vi "ConfigureDlg.vi"(8 "error in (no error)":errorcluster, 11 "C37.118 PMU in":refnum<class "C37.118 Sim.lvclass">) -> (0 "error out":errorcluster, 2 "Changed":bool, 3 "C37.118 PMU out":refnum<class "C37.118 Sim.lvclass">)   [LabVIEW 2018, in "SensorPlugins.lvlib" / "C37.118 Sim.lvclass"]
uses:
  C37.118 Sim.lvclass
  X:/Projects/PMUCal/Modules/Sensor/SensorPlugins/PmuBaseClass/PmuBase.lvclass
  C:/Program Files (x86)/National Instruments/LabVIEW 2018/user.lib/NIST/BaseClasses/BasePlugin_class/BasePlugin.lvclass
  PmuBaseClass/Typedef/PmuConfig.ctl
  PmuBaseClass/Typedef/ePhases.ctl
  PmuBaseClass/PmuBase.lvclass/PmuBase.ctl
  C37.118 Sim.lvclass/C37.118 Sim.ctl
  <userlib>/NIST/BaseClasses/BasePlugin_class/BasePlugin.lvclass/BasePlugin.ctl
  FGen/MemberClasses/FunctionBaseClass/FunctionBase.lvclass
  PmuBaseClass/Accessors/Read PmuConfig.vi
  PmuBaseClass/Accessors/Read PhaseArray.vi
  Accessors/Read FunctionIniFilePath.vi
  PmuBaseClass/Accessors/Write PmuConfig.vi
  PmuBaseClass/Accessors/Write PhaseArray.vi
  <userlib>/NIST/BaseClasses/BasePlugin_class/Accessors/Read PluginIniFilePath.vi
  <userlib>/NIST/BaseClasses/BasePlugin_class/Accessors/Write PluginIniFilePath.vi
  Accessors/Write Function.vi
  Accessors/Write FunctionIniFilePath.vi
  Accessors/Read Function.vi
  <vilib>/Utility/error.llb/Error Cluster From Error Code.vi
  <vilib>/ErrorRing/Error Ring.xnode
  <vilib>/Utility/config.llb/NI_LVConfig.lvlib
  <userlib>/NIST/NISTErrorLib/NISTErrorLib.lvlib
  <userlib>/NIST/BaseClasses/Object_class/BaseObject.lvclass
  PmuBaseClass/PmuBase.lvclass
panel:
  in  "btnSaveAs":bool
  in  "FunctionIniFilePath":path
  in  "btnFuncConfig":bool
  in  "btnCancel":bool
  in  "BtnDone":bool
  in  "PhaseArray":T1[](array[typedef])=[enum."VA", enum."VB", enum."VC", enum."V+", enum."IA", enum."IB", enum."IC", enum."I+"]
  in  "PmuConfig":T2={"Class"=enum."M", "Fs"=60, "F0"=60, "FSamp"=60, "SettlingTime"=0.0, "T0"=0.0}
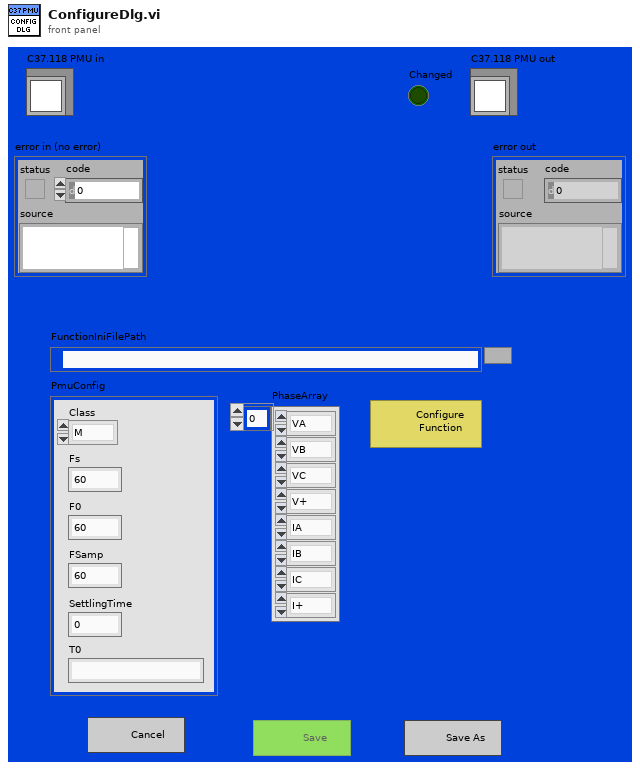
[diagram p1: front panel]
types:
  T1 = typedef "SensorPlugins.lvlib/PmuBase.lvclass/ePhases.ctl" = enum16{"VA", "VB", "VC", "V+", "IA", "IB", "IC", "I+", "none"}
  T2 = typedef "SensorPlugins.lvlib/PmuBase.lvclass/PmuConfig.ctl" = cluster{"Class":enum16{"M", "P"}, "Fs":i32, "F0":i32, "FSamp":i32, "SettlingTime":dbl, "T0":ext}
  T3 = enum8{"Enabled", "Disabled", "Disabled and Grayed Out"}
  T4 = enum32{"Invalid", "Standard", "Closed", "Hidden", "Minimized", "Maximized"}
  T5 = enum32{"Invalid", "Default", "Floating", "Floating/Auto-Hide", "Modal"}
  T6 = typedef "NI_LVConfig.lvlib/Config Data RefNum.ctl" = refnum<k1>
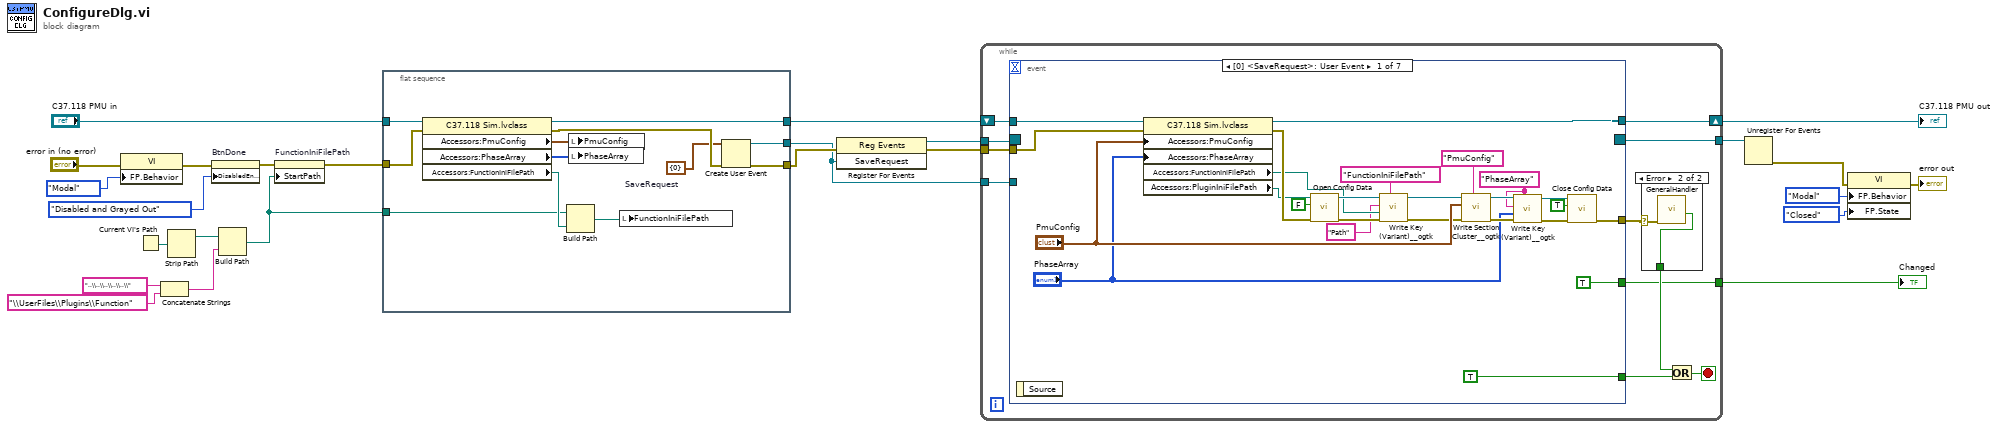
[diagram p0: block diagram]
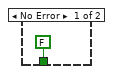
[diagram p2: hidden frame]
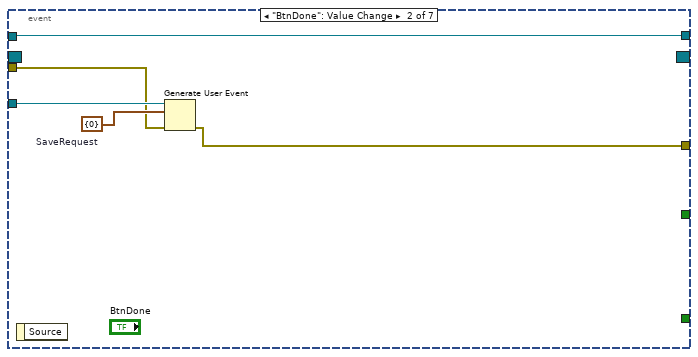
[diagram p3: hidden frame]
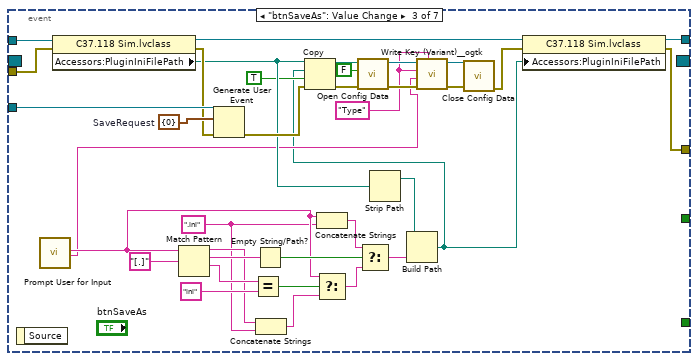
[diagram p4: hidden frame]
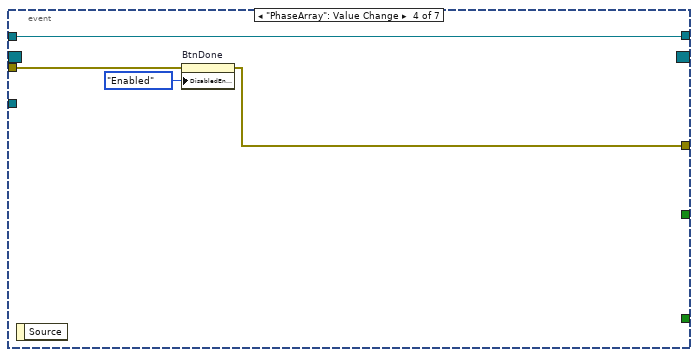
[diagram p5: hidden frame]
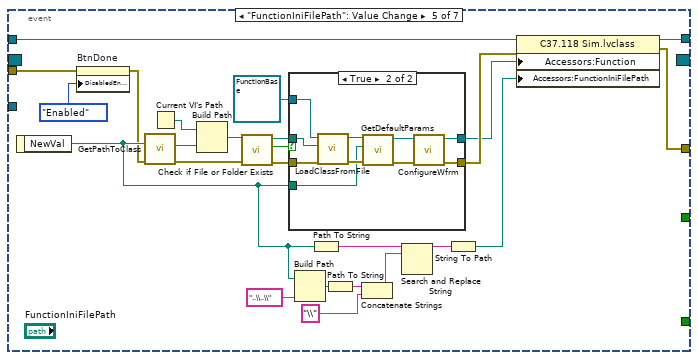
[diagram p6: hidden frame]
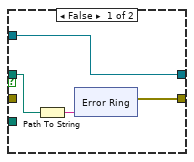
[diagram p7: hidden frame]
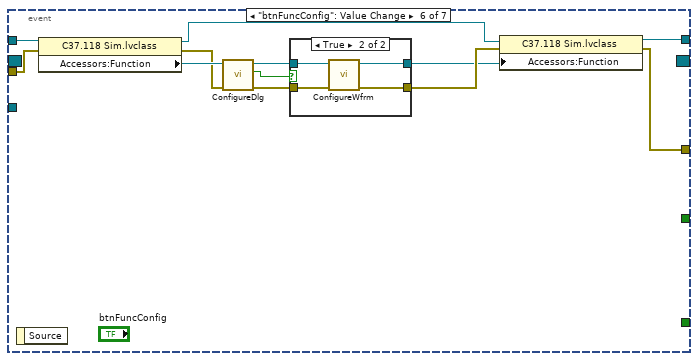
[diagram p8: hidden frame]
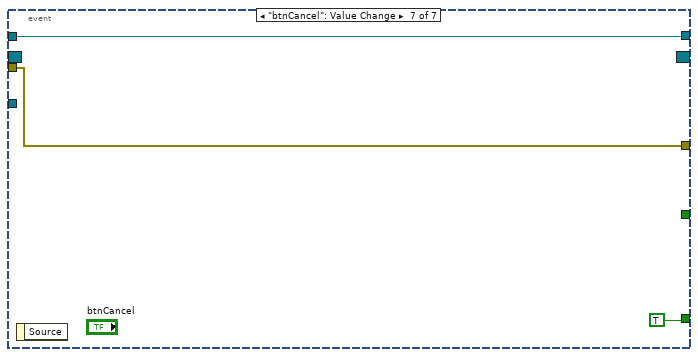
[diagram p10: hidden frame]
diagram:
  n1 = property class="VI"(error in="error in (no error)", "FP.Behavior"=T5."Modal" ("Front Panel Window:Behavior")) -> (error out=w16:errorcluster)  [unwired: 1 in, 1 out]
  n2 = Current VI's Path() -> (path=w11:path)
  n3 = Concatenate Strings("..\\..\\..\\..\\..\\", "\\UserFiles\\Plugins\\Function" ("name or relative path")) -> (w13:string)
  n4 = Strip Path(path=w11) -> (stripped path=w14:path)  [unwired: 1 out]
  n5 = property on="BtnDone" class="Bool"(error in=w16, "DisabledEnum"=T3."Disabled and Grayed Out" ("Disabled")) -> (error out=w9:errorcluster)  [unwired: 1 in, 1 out]
  n6 = Build Path(base path=w14, name or relative path=w13) -> (appended path=w7:path)
  n7 = property on="FunctionIniFilePath" class="Path"(error in=w9, "StartPath"=w7) -> (error out=w8:errorcluster)  [unwired: 1 in, 1 out]
  n8 = flat-sequence {
    tunnel: "C37.118 PMU in" -> [w37]
    tunnel: [w36] -> w23
    tunnel: [w29] -> w6
    tunnel: w8 -> [w35]
    tunnel: w7 -> [w31]
    tunnel: [w26] -> w4
    frame #0 {
      w27 = cluster{"Num":i32} {"Num"=0}  # SaveRequest
      n9 = property class="C37.118 Sim.lvclass"(reference=w37, error in=w35) -> (reference out=w36:refnum<class "C37.118 Sim.lvclass">, error out=w28:errorcluster, "Accessors:PmuConfig"=w34:T2, "Accessors:PhaseArray"=w33:T1[], "Accessors:FunctionIniFilePath"=w32:path)
      n10 = Build Path(base path=w31, name or relative path=w32) -> (appended path=w30:path)
      n11 = local write "PmuConfig"(w34) -> ()
      n12 = local write "PhaseArray"(w33) -> ()
      n13 = local write "FunctionIniFilePath"(w30) -> ()
      n14 = Create User Event(user event datatype=w27, error in=w28) -> (user event=w26:refnum<user-event>, error out=w29:errorcluster)
    }
  }
  n15 = register-events(error in=w6, w4) -> (reference out=w3:refnum<event-registration>, error out=w5:errorcluster)  [unwired: 1 in]
  n16 = while {
    shift-right: [w46] -> w24
    shift-left: w23 -> [w48]
    tunnel: w5 -> [w47]
    tunnel: [w41] -> w21
    tunnel: w4 -> [w40]
    tunnel: w3 -> [w39]
    tunnel: [w38] -> w2
    stop <- w42 stop-if-true
    n17 = event shown="[0] <SaveRequest>: User Event" {
      selector: w39 -> [_ _ _ _ _ _ _]
      dyn-events: [_ _ _ _ _ _ _] -> w38
      timeout: _ -> [_ _ _ _ _ _ _]
      tunnel: w48 -> [w76 w77 w105 w120 w131 w179 w188]
      tunnel: w47 -> [w74 w79 w102 w121 w124 w178 w187]
      tunnel: [w63 w78 w83 w118 w125 w173 w187] -> w43
      tunnel: [TRUE _ _ _ _ _ TRUE] -> w45
      tunnel: [w73 w77 w103 w120 w126 w174 w188] -> w46
      tunnel: [TRUE _ _ _ _ _ _] -> w41
      tunnel: w40 -> [_ w81 w101 _ _ _ _]
      event User Event {
        w62 = "PhaseArray" ("section (optional)")
        n18 = event-data() -> ()  [unwired: 1 in, 1 out]
        n19 = property class="C37.118 Sim.lvclass"(reference=w76, error in=w74, "Accessors:PmuConfig"="PmuConfig", "Accessors:PhaseArray"="PhaseArray") -> (reference out=w73:refnum<class "C37.118 Sim.lvclass">, error out=w71:errorcluster, "Accessors:FunctionIniFilePath"=w53:path, "Accessors:PluginIniFilePath"=w58:path)
        n20 = call <vilib>:"Open Config Data.vi"("error in (no error)"=w71, "create file if necessary (T)"=FALSE, "configuration file path"=w58) -> ("error out"=w56:errorcluster, "refnum"=w70:T6)  [unwired: 6 in, 1 out]
        n21 = call <userlib>:"Write Key (Variant)__ogtk.vi"("section"="FunctionIniFilePath", "error in (no error)"=w56, "key-value"=w53, "key (optional)"="Path", "refnum"=w70) -> ("error out"=w55:errorcluster, "refnum out"=w57:T6)  [unwired: 5 in]
        n22 = call <userlib>:"Write Section Cluster__ogtk.vi"("section (optional)"="PmuConfig", "error in (no error)"=w55, "Section Formatted Cluster"="PmuConfig", "refnum"=w57) -> ("error out"=w67:errorcluster, "dup refnum"=w66:T6)  [unwired: 6 in]
        n23 = call <userlib>:"Write Key (Variant)__ogtk.vi"("section"=w62, "error in (no error)"=w67, "key-value"="PhaseArray", "key (optional)"=w62, "refnum"=w66) -> ("error out"=w60:errorcluster, "refnum out"=w61:T6)  [unwired: 5 in]
        n24 = call <vilib>:"Close Config Data.vi"("error in (no error)"=w60, "write file if changed (T)"=TRUE, "refnum"=w61) -> ("error out"=w63:errorcluster)  [unwired: 7 in, 1 out]
      }
      event "BtnDone": Value Change {
        w80 = cluster{"Num":i32} {"Num"=0}  # SaveRequest
        n25 = event-data() -> ()  [unwired: 1 in, 1 out]
        n26 = Generate User Event(user event=w81, event data cluster=w80, error in=w79) -> (error out=w78:errorcluster)  [unwired: 1 in, 1 out]
      }
      event "btnSaveAs": Value Change {
        w82 = "Type"
        w100 = cluster{"Num":i32} {"Num"=0}  # SaveRequest
        w86 = ".ini" ("string")
        n27 = event-data() -> ()  [unwired: 1 in, 1 out]
        n28 = call "Prompt User for Input"() -> ("File Name"=w106:string, "PluginType Name"=w87:string)  [unwired: 16 in, 2 out]
        n29 = property class="C37.118 Sim.lvclass"(reference=w105, error in=w102) -> (reference out=w104:refnum<class "C37.118 Sim.lvclass">, error out=w99:errorcluster, "Accessors:PluginIniFilePath"=w90:path)
        n30 = Match Pattern(string=w106, regular expression="[.]" ("string")) -> (before substring=w113:string, match substring=w115:string, after substring=w116:string)  [unwired: 1 in, 1 out]
        n31 = Generate User Event(user event=w101, event data cluster=w100, error in=w99) -> (error out=w91:errorcluster)  [unwired: 1 in, 1 out]
        n32 = Equal?(x=w116, y="ini" ("string")) -> (x = y?=w112:bool)
        n33 = Empty String/Path?(string/path=w115) -> (empty?=w110:bool)
        n34 = Concatenate Strings(w113, w86) -> (w111:string)
        n35 = Concatenate Strings(w106, w86) -> (w108:string)
        n36 = Select(t=w106, s=w112, f=w111) -> (s? t:f=w109:string)
        n37 = Select(t=w108, s=w110, f=w109) -> (s? t:f=w107:string)
        n38 = Strip Path(path=w90) -> (stripped path=w89:path)  [unwired: 1 out]
        n39 = Build Path(base path=w89, name or relative path=w107) -> (appended path=w85:path)
        n40 = Copy(8:w91, 9:TRUE ("overwrite (F)"), 10:w85, 11:w90) -> (0:w92:errorcluster, 3:w93:path)  [unwired: 1 in, 1 out]
        n41 = call <vilib>:"Open Config Data.vi"("error in (no error)"=w92, "create file if necessary (T)"=FALSE, "configuration file path"=w93) -> ("error out"=w95:errorcluster, "refnum"=w96:T6)  [unwired: 6 in, 1 out]
        n42 = call <userlib>:"Write Key (Variant)__ogtk.vi"("section"=w82, "error in (no error)"=w95, "key-value"=w87, "key (optional)"=w82, "refnum"=w96) -> ("error out"=w97:errorcluster, "refnum out"=w98:T6)  [unwired: 5 in]
        n43 = call <vilib>:"Close Config Data.vi"("error in (no error)"=w97, "refnum"=w98) -> ("error out"=w84:errorcluster)  [unwired: 8 in, 1 out]
        n44 = property class="C37.118 Sim.lvclass"(reference=w104, error in=w84, "Accessors:PluginIniFilePath"=w85) -> (reference out=w103:refnum<class "C37.118 Sim.lvclass">, error out=w83:errorcluster)
      }
      event "PhaseArray": Value Change {
        n45 = event-data() -> ()  [unwired: 1 in, 1 out]
        n46 = property on="BtnDone" class="Bool"(error in=w121, "DisabledEnum"=T3."Enabled" ("Disabled")) -> (error out=w118:errorcluster)  [unwired: 1 in, 1 out]
      }
      event "FunctionIniFilePath": Value Change {
        n47 = event-data() -> ("NewVal"=w132:path)  [unwired: 1 in]
        n48 = property on="BtnDone" class="Bool"(error in=w124, "DisabledEnum"=T3."Enabled" ("Disabled")) -> (error out=w123:errorcluster)  [unwired: 1 in, 1 out]
        n49 = call <userlib>:"GetPathToClass.vi"("error in (no error)"=w123, "configuration file path"=w132) -> ("error IO"=w143:errorcluster, "PathToClass"=w146:path)  [unwired: 8 in]
        n50 = Current VI's Path() -> (path=w145:path)
        n51 = Build Path(base path=w145, name or relative path=w146) -> (appended path=w144:path)
        n52 = call <vilib>:"Check if File or Folder Exists.vi"("error in (no error)"=w143, "path"=w144) -> ("error out"=w140:errorcluster, "file or folder exists?"=w142:bool, "dup path"=w141:path)  [unwired: 7 in]
        n53 = case shown="True" w142 {
          tunnel: w141 -> [w149 w167]
          tunnel: w140 -> [_ w165]
          tunnel: refnum<class "FunctionBase.lvclass"> refnum ("Functions.lvlib:FunctionBase.lvclass") -> [w147 w166]
          tunnel: w132 -> [_ w162]
          tunnel: [w148 w161] -> w130
          tunnel: [w147 w160] -> w129
          frame False {
            n54 = Path To String(path=w149) -> (string=w150:string)
            n55 = xnode "Error Ring"("parameter 0"=w150) -> ("error out"=w148:errorcluster)
          }
          frame True {
            n56 = call-dynamic "LoadClassFromFile.vi"("error in (no error)"=w165, "class path"=w167, "reference in"=w166) -> ("error out"=w164:errorcluster, "reference out"=w163:refnum<class "FunctionBase.lvclass">)  [unwired: 7 in]
            n57 = call-dynamic "GetDefaultParams.vi"("error in (no error)"=w164, "Path"=w162, "FunctionBase in"=w163) -> ("error out"=w158:errorcluster, "FunctionBase out"=w159:refnum<class "FunctionBase.lvclass">)  [unwired: 7 in]
            n58 = call-dynamic "ConfigureWfrm.vi"("error in (no error)"=w158, "FunctionBase in"=w159) -> ("error out"=w161:errorcluster, "FunctionBase out"=w160:refnum<class "FunctionBase.lvclass">)  [unwired: 8 in]
          }
        }
        n59 = Build Path(base path=w132, name or relative path="..\\..\\") -> (appended path=w136:path)
        n60 = Path To String(path=w132) -> (string=w137:string)
        n61 = Path To String(path=w136) -> (string=w135:string)
        n62 = Concatenate Strings(w135, "\\" ("string")) -> (w133:string)
        n63 = Search and Replace String(input string=w137, search string=w133) -> (result string=w128:string)  [unwired: 6 in, 3 out]
        n64 = String To Path(string=w128) -> (path=w127:path)
        n65 = property class="C37.118 Sim.lvclass"(reference=w131, error in=w130, "Accessors:Function"=w129, "Accessors:FunctionIniFilePath"=w127) -> (reference out=w126:refnum<class "C37.118 Sim.lvclass">, error out=w125:errorcluster)
      }
      event "btnFuncConfig": Value Change {
        n66 = event-data() -> ()  [unwired: 1 in, 1 out]
        n67 = property class="C37.118 Sim.lvclass"(reference=w179, error in=w178) -> (reference out=w175:refnum<class "C37.118 Sim.lvclass">, error out=w176:errorcluster, "Accessors:Function"=w177:refnum<class "FunctionBase.lvclass">)
        n68 = call-dynamic "ConfigureDlg.vi"("error in (no error)"=w176, "FunctionBase in"=w177) -> ("error out"=w171:errorcluster, "Changed"=w168:bool, "FunctionBase out"=w172:refnum<class "FunctionBase.lvclass">)  [unwired: 7 in]
        n69 = case shown="True" w168 {
          tunnel: w172 -> [w181 w185]
          tunnel: w171 -> [w180 w184]
          tunnel: [w180 w183] -> w170
          tunnel: [w181 w182] -> w169
          frame False {
          }
          frame True {
            n70 = call-dynamic "ConfigureWfrm.vi"("error in (no error)"=w184, "FunctionBase in"=w185) -> ("error out"=w183:errorcluster, "FunctionBase out"=w182:refnum<class "FunctionBase.lvclass">)  [unwired: 8 in]
          }
        }
        n71 = property class="C37.118 Sim.lvclass"(reference=w175, error in=w170, "Accessors:Function"=w169) -> (reference out=w174:refnum<class "C37.118 Sim.lvclass">, error out=w173:errorcluster)
      }
      event "btnCancel": Value Change {
        n72 = event-data() -> ()  [unwired: 1 in, 1 out]
      }
    }
    n73 = case shown="Error" w43 {
      selector: w43 -> [_ w50]
      tunnel: [FALSE ("Stop") w51] -> w44
      frame No Error {
      }
      frame Error {
        n74 = call <userlib>:"GeneralHandler.vi"("error in (no error)"=w50) -> ("Stop"=w51:bool)  [unwired: 7 in, 3 out]
      }
    }
    n75 = Or(x=w44, y=w45) -> (x .or. y?=w42:bool)
  }
  "C37.118 PMU out" <- w24
  "Changed" <- w21
  n76 = Unregister For Events(event registration refnum=w2) -> (error out=w1:errorcluster)  [unwired: 1 in]
  n77 = property class="VI"(error in=w1, "FP.Behavior"=T5."Modal" ("Front Panel Window:Behavior"), "FP.State"=T4."Closed" ("Front Panel Window:State")) -> (error out=→"error out":errorcluster)  [unwired: 1 in, 1 out]
